vi "Meta Data Error Check.vi"(8 "error in (no error)":errorcluster, 10 "Voltage Level (0V)":dbl, 11 "Meta Data":string[][](array[string])) -> (0 "error out":errorcluster, 3 "No Error":bool)   [LabVIEW 2013]
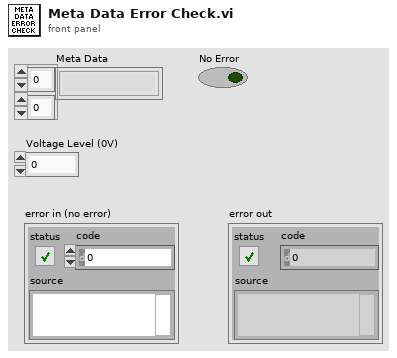
[diagram p1: front panel]
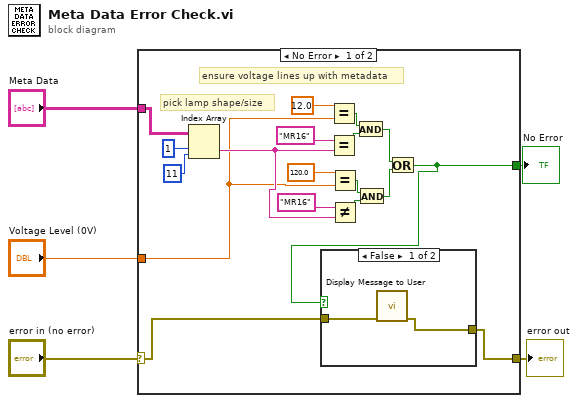
[diagram p0: block diagram]
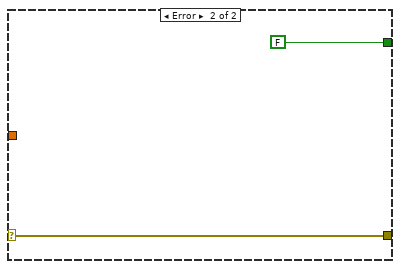
[diagram p3: hidden frame]
diagram:
  n1 = case shown="No Error" "error in (no error)" {
    selector: "error in (no error)" -> [w8 w28]
    tunnel: [w6 FALSE] -> w5
    tunnel: "Voltage Level (0V)" -> [w9 _]
    tunnel: "Meta Data" -> [w10 _]
    tunnel: [w7 w28] -> w1
    frame No Error {
      # "pick lamp shape/size"
      # "ensure voltage lines up with metadata"
      n2 = Index Array(array=w10, index (row)=1 ("disabled index (row)"), index (col)=11 ("disabled index (col)")) -> (element=w21:string)
      n3 = Equal?(x=12.0, y=w9) -> (x = y?=w15:bool)
      n4 = Equal?(x="MR16", y=w21) -> (x = y?=w16:bool)
      n5 = Equal?(x=120.0, y=w9) -> (x = y?=w18:bool)
      n6 = Not Equal?(x="MR16", y=w21) -> (x != y?=w17:bool)
      n7 = And(x=w15, y=w16) -> (x .and. y?=w22:bool)
      n8 = And(x=w18, y=w17) -> (x .and. y?=w23:bool)
      n9 = Or(x=w22, y=w23) -> (x .or. y?=w6:bool)
      n10 = case shown="False" w6 {
        tunnel: w8 -> [w25 w26]
        tunnel: [w24 w26] -> w7
        frame False {
          n11 = call "Display Message to User"("error in (no error)"=w25) -> ("error out"=w24:errorcluster)  [unwired: 9 in, 1 out]
        }
        frame True {
        }
      }
    }
    frame Error {
    }
  }
  "No Error" <- w5
  "error out" <- w1
